vi "getXMLAcquisitionParameters.vi"(8 "error in":errorcluster, 9 "usb/RS170":bool, 11 "Axquisition Parameters Node":refnum<k20>) -> (0 "error out":errorcluster, 3 "Acquisition Parameters":T1={"Brightness"=0.0, "Contrast"=1.0, "Saturation"=1.0, "White level"=0.7} {"White level" scale=0.3..1.26 scale format="%#_2f"; "Saturation" scale=0.5..1.5 scale format="%#_3f"; "Contrast" scale=0.4..1.5 scale format="%#_3f"; "Brightness" scale=-50.0..50.0 scale format="%#_2f"})   [LabVIEW 2013]
uses:
  <vilib>/xml/NI_XML.lvlib
panel:
  out "error out 2":errorcluster
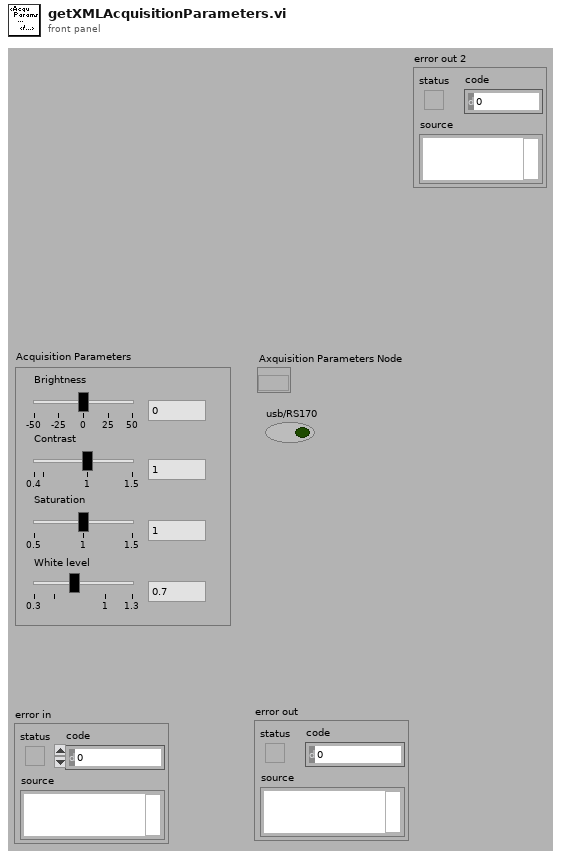
[diagram p1: front panel]
types:
  T1 = cluster{"Brightness":dbl, "Contrast":dbl, "Saturation":dbl, "White level":dbl}
  T2 = cluster{"[0]":dbl, "[1]":dbl, "[2]":dbl, "[3]":dbl, "[4]":dbl, "[5]":dbl, "[6]":dbl, "[7]":dbl, "[8]":dbl}
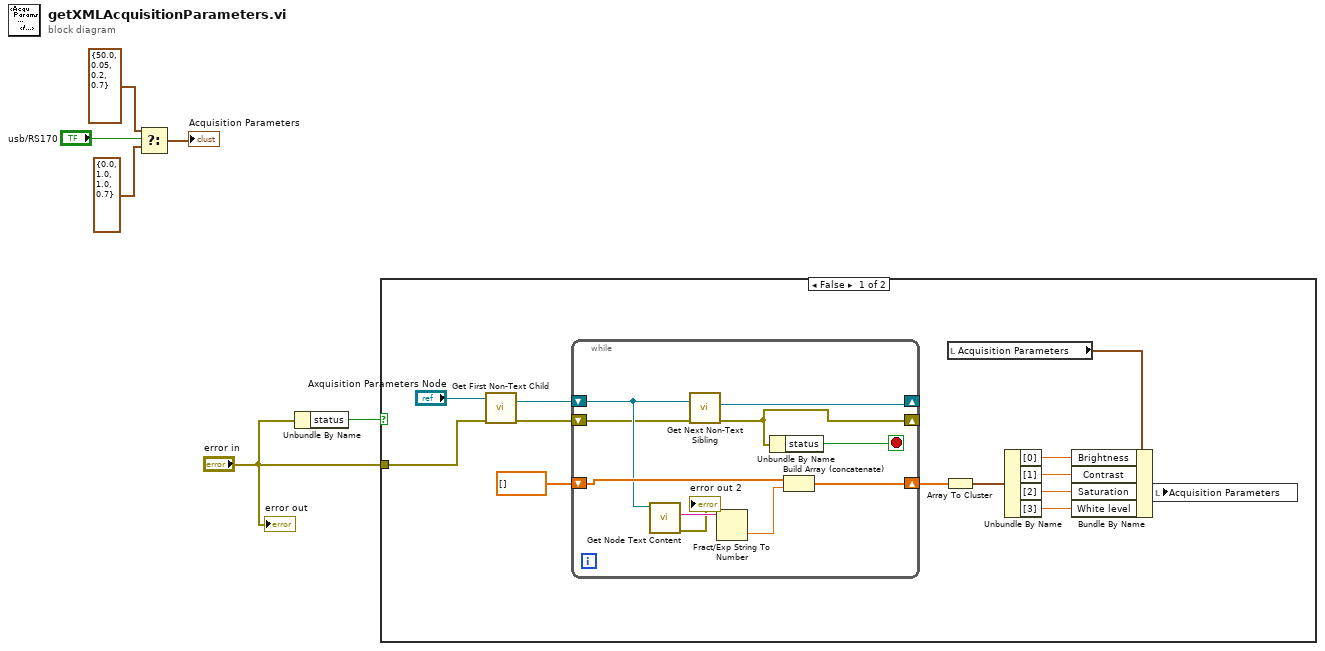
[diagram p0: block diagram]
diagram:
  n1 = Select(t=T1 {"Brightness"=50.0, "Contrast"=0.05, "Saturation"=0.2, "White level"=0.7} ("Acquisition Parameters"), s="usb/RS170", f=T1 {"Brightness"=0.0, "Contrast"=1.0, "Saturation"=1.0, "White level"=0.7} ("Acquisition Parameters")) -> (s? t:f=→"Acquisition Parameters":T1)
  n2 = Unbundle By Name("error in") -> ("status"=w6:bool)
  n3 = case shown="False" w6 {
    tunnel: "error in" -> [w9 _]
    frame False {
      n4 = call <vilib>:"Get First Non-Text Child.vi"("error in (no error)"=w9, "node in"="Axquisition Parameters Node") -> ("error out"=w7:errorcluster, "child node"=w8:refnum<k20>)  [unwired: 6 in, 2 out]
      n5 = while {
        shift-right: [w22] -> _
        shift-left: w8 -> [w24]
        shift-right: [w21] -> _
        shift-left: w7 -> [w23]
        shift-right: [w27] -> w18
        shift-left: dbl[] [] -> [w25]
        stop <- w28 stop-if-true
        n6 = call <vilib>:"Get Node Text Content.vi"("node in"=w24) -> ("error out"=→"error out 2":errorcluster, "node text"=w29:string)  [unwired: 8 in, 1 out]
        n7 = call <vilib>:"Get Next Non-Text Sibling.vi"("error in (no error)"=w23, "node in"=w24) -> ("error out"=w21:errorcluster, "sibling node"=w22:refnum<k20>)  [unwired: 6 in, 2 out]
        n8 = Fract/Exp String To Number(string=w29) -> (number=w26:dbl)  [unwired: 3 in, 1 out]
        n9 = Unbundle By Name(w21) -> ("status"=w28:bool)
        n10 = Build Array (concatenate)(w25, w26) -> (w27:dbl[])
      }
      n11 = Array To Cluster(array=w18) -> (cluster=w17:T2)
      n12 = local read "Acquisition Parameters"() -> (w16:T1)
      n13 = Unbundle By Name(w17) -> ("[0]"=w15:dbl, "[1]"=w14:dbl, "[2]"=w13:dbl, "[3]"=w12:dbl)
      n14 = Bundle By Name(cluster=w16, "Brightness"=w15, "Contrast"=w14, "Saturation"=w13, "White level"=w12) -> (w11:T1)
      n15 = local write "Acquisition Parameters"(w11) -> ()
    }
    frame True {
    }
  }
  "error out" <- "error in"
